vi "Configure Modulation Waveform (Dual-Sine).vi"(7 "Modulation Path (1)":u16(ring)=1 items=["1"=1, "2"=2], 8 "error in (no error)":errorcluster, 9 "Tone2 Amplitude Percent (50 percent)":dbl=50.0, 10 "Modulation Type (0: Amplitude Modulation)":u16(ring) items=["Amplitude Modulation", "Frequency Modulation", "Phase Modulation", "Low Frequency Output"], 11 "VISA resource name":refnum<visa-resource-name>) -> (0 "error out":errorcluster, 3 "VISA resource name out":refnum<visa-resource-name>)   [LabVIEW 2009, in "Agilent PSG MXG Series.lvlib"]
doc: "Configures the amplitude of the second tone for a dual-sine waveform as a percentage of the total amplitude.\n\n<B>Notes:</B>\n(1) This VI is <B>NOT</B> valid in E8247C, N5181A, N5182A, N5183A.\n\n(2) For E8257D, E8267D, this VI is valid only when the instrument installs <B>Option UNT</B> (AM, FM, phase modulation, and LF output)."
uses:
  Agilent PSG MXG Series.lvlib
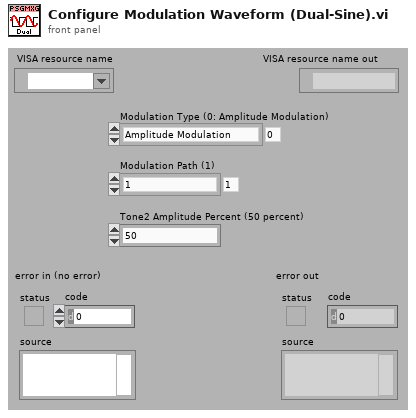
[diagram p1: front panel]
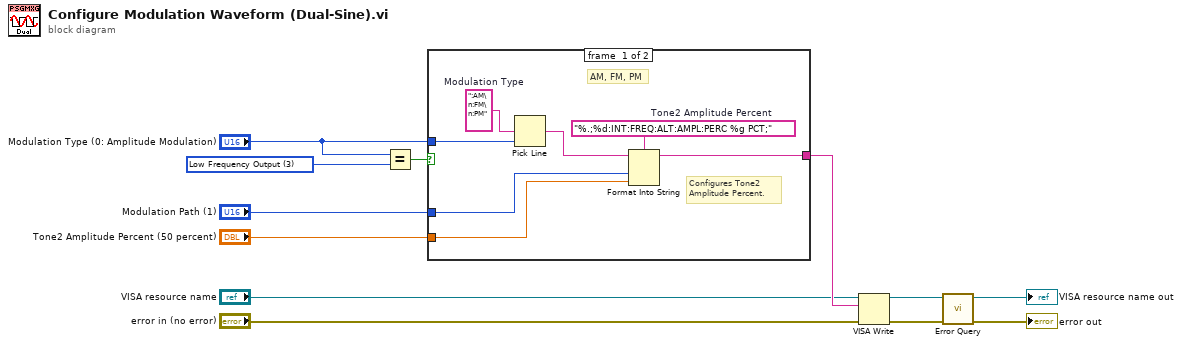
[diagram p0: block diagram]
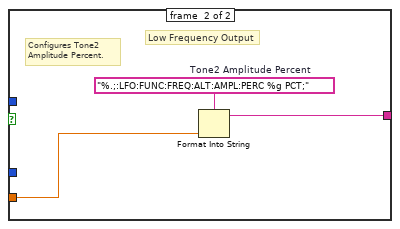
[diagram p2: hidden frame]
diagram:
  w7 = u16 3 items=["Amplitude Modulation", "Frequency Modulation", "Phase Modulation", "Low Frequency Output"] ("Modulation Type (0: Amplitude Modulation)")
  n1 = Equal?(x="Modulation Type (0: Amplitude Modulation)", y=w7) -> (x = y?=w12:bool)
  n2 = case shown="False" w12 {
    tunnel: "Modulation Type (0: Amplitude Modulation)" -> [w16 _]
    tunnel: "Modulation Path (1)" -> [w15 _]
    tunnel: "Tone2 Amplitude Percent (50 percent)" -> [w14 w21]
    tunnel: [w13 w20] -> w11
    frame #0 {
      w18 = "%.;%d:INT:FREQ:ALT:AMPL:PERC %g PCT;"  # Tone2 Amplitude Percent
      w19 = ":AM\n:FM\n:PM"  # Modulation Type
      # "Configures Tone2\nAmplitude Percent."
      # "AM, FM, PM"
      n3 = Pick Line(multi-line string=w19, line index=w16) -> (output string=w17:string)  [unwired: 1 out]
      n4 = Format Into String(format string=w18, initial string=w17, w15, w14) -> (resulting string=w13:string)  [unwired: 1 in, 1 out]
    }
    frame #1 {
      w22 = "%.;:LFO:FUNC:FREQ:ALT:AMPL:PERC %g PCT;"  # Tone2 Amplitude Percent
      # "Configures Tone2\nAmplitude Percent."
      # "Low Frequency Output"
      n5 = Format Into String(format string=w22, w21) -> (resulting string=w20:string)  [unwired: 2 in, 1 out]
    }
  }
  n6 = VISA Write(VISA resource name="VISA resource name", write buffer=w11, error in (no error)="error in (no error)") -> (VISA resource name out=w10:refnum<visa-resource-name>, error out=w9:errorcluster)  [unwired: 1 out]
  n7 = call "Error Query.vi"("error in (no error)"=w9, "VISA resource name"=w10) -> ("error out"=→"error out":errorcluster, "VISA resource name out"=→"VISA resource name out":refnum<visa-resource-name>)  [unwired: 8 out]
